vi "Read EDS File.vi"(8 "error in":errorcluster, 10 "EDS File Path":path, 11 "UI Actor in":refnum<class "UI Actor.lvclass">) -> (0 "error out":errorcluster, 3 "UI Actor out":refnum<class "UI Actor.lvclass">)   [LabVIEW 2024, in "UI Actor.lvlib" / "UI Actor.lvclass"]
uses:
  UI Actor.lvclass
  Core/EDS/EDS.lvclass
  Core/EDS/EDS.lvclass/EDS.ctl
  UI Actor.lvclass/UI Actor.ctl
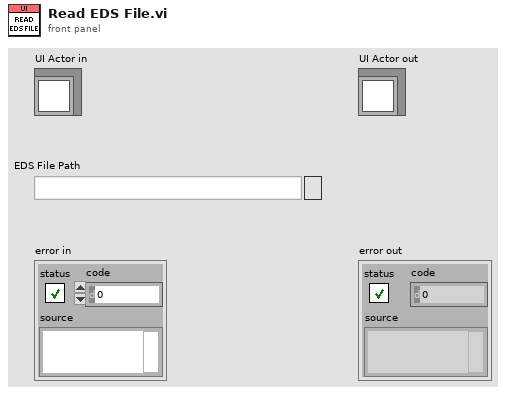
[diagram p1: front panel]
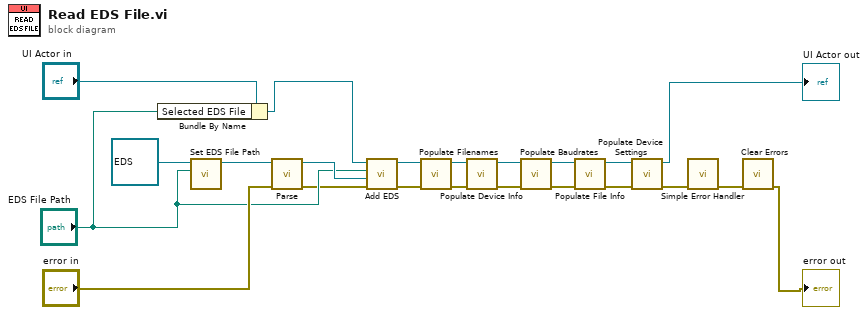
[diagram p0: block diagram]
diagram:
  n1 = Bundle By Name(cluster="UI Actor in", "Selected EDS File"="EDS File Path") -> (w9:refnum<class "UI Actor.lvclass">)
  n2 = call "Set EDS File Path.vi"("EDS File Path"="EDS File Path", "EDS in"=refnum<class "EDS.lvclass"> refnum) -> ("EDS out"=w21:refnum<class "EDS.lvclass">)  [unwired: 9 in]
  n3 = call "Parse.vi"("error in"="error in", "EDS in"=w21) -> ("error out"=w7:errorcluster, "EDS out"=w17:refnum<class "EDS.lvclass">)  [unwired: 8 in]
  n4 = call "Add EDS.vi"("EDS"=w17, "File Path"="EDS File Path", "UI Actor in"=w9) -> ("UI Actor out"=w5:refnum<class "UI Actor.lvclass">)  [unwired: 8 in]
  n5 = call "Populate Filenames.vi"("error in"=w7, "UI Actor in"=w5) -> ("error out"=w6:errorcluster, "UI Actor out"=w4:refnum<class "UI Actor.lvclass">)  [unwired: 8 in]
  n6 = call "Populate Device Info.vi"("error in"=w6, "UI Actor in"=w4) -> ("error out"=w16:errorcluster, "UI Actor out"=w14:refnum<class "UI Actor.lvclass">)  [unwired: 8 in]
  n7 = call "Populate Baudrates.vi"("error in"=w16, "UI Actor in"=w14) -> ("error out"=w15:errorcluster, "UI Actor out"=w12:refnum<class "UI Actor.lvclass">)  [unwired: 8 in]
  n8 = call "Populate File Info.vi"("error in"=w15, "UI Actor in"=w12) -> ("error out"=w13:errorcluster, "UI Actor out"=w11:refnum<class "UI Actor.lvclass">)  [unwired: 8 in]
  n9 = call "Populate Device Settings.vi"("error in"=w13, "UI Actor in"=w11) -> ("error out"=w20:errorcluster, "UI Actor out"=→"UI Actor out":refnum<class "UI Actor.lvclass">)  [unwired: 8 in]
  n10 = call <vilib>:"Simple Error Handler.vi"("error in (no error)"=w20) -> ("error out"=w3:errorcluster)  [unwired: 4 in, 4 out]
  n11 = call <vilib>:"Clear Errors.vi"("error in (no error)"=w3) -> ("error out"=→"error out":errorcluster)  [unwired: 5 in, 1 out]
